vi "pcadctest.vi"() -> ()   [LabVIEW 2022 SP3]
uses:
  <vilib>/MakerHub/LINX/Public/Utilities/Open Serial.vi
  PCA/PCA.lvclass
  <vilib>/MakerHub/LINX/LMH-LINX.lvlib
panel:
  in  "Val 2 off":u16
  in  "Val off":u16
  in  "Val 3":u16=4095 format="%b"
  in  "Val 2":u16
  in  "Val":u16
  in  "GO":bool
  out "error out":errorcluster
  in  "stop":bool
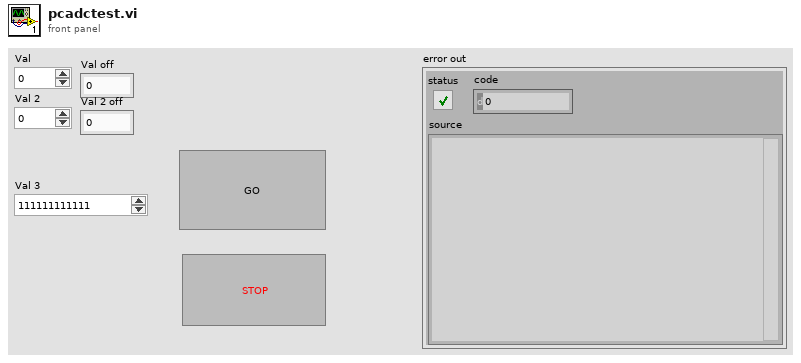
[diagram p1: front panel]
types:
  T1 = typedef "LMH-LINX.lvlib/LINX Ref.ctl" = cluster{"IO":T2, "Interface":T3, "LINX Device Config":T4}
  T2 = typedef "LMH-LINX.lvlib/Platform.ctl" = enum16{"Remote", "Local"}
  T3 = typedef "LMH-LINX.lvlib/Interface.ctl" = enum16{"Serial", "TCP"}
  T4 = typedef "LMH-LINX.lvlib/Device.lvlib/LINX Device Config.ctl" = cluster{"Interface":T3, "COM Port":refnum<visa-resource-name>, "TCP Configuration":T5, "Device Family":u8, "Device ID":u8, "Device Name":string, "TCP Ref":refnum<k5>, "Channels":T6}
  T5 = typedef "LMH-LINX.lvlib/Device.lvlib/TCP Config.ctl" = cluster{"IP Address":string, "Port":u16}
  T6 = typedef "LMH-LINX.lvlib/Channels.ctl" = cluster{"DI":u8[], "DO":u8[], "AI":u8[], "AO":u8[], "PWM":u8[], "QE":u8[], "UART":u8[], "I2C 2":u8[], "SPI":u8[], "CAN":u8[], "Servo":u8[], "AI Ref (V)":dbl, "AI Resolution (Bits)":u8, "AO Ref (V)":dbl, "AO Resolution (Bits)":u8}
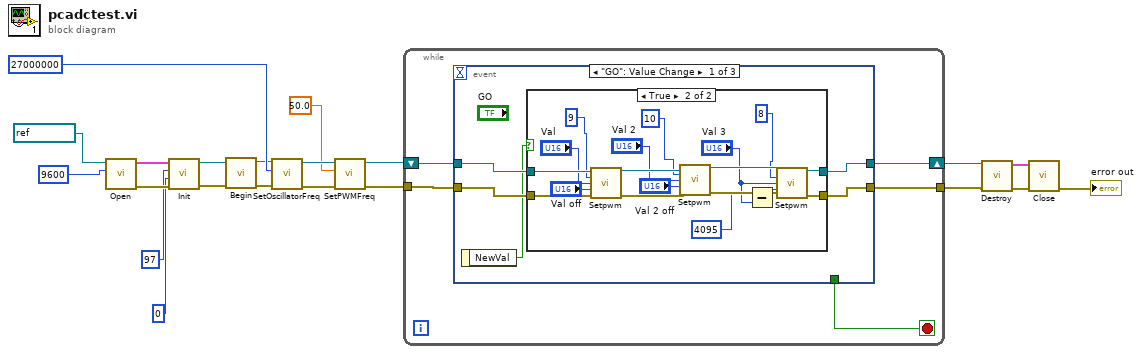
[diagram p0: block diagram]
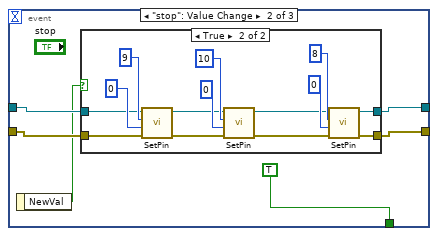
[diagram p3: hidden frame]
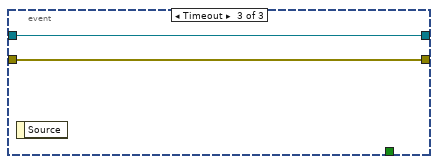
[diagram p5: hidden frame]
diagram:
  n1 = call-poly <vilib>:"Open.vi"("Baud Rate Override"=u32 9600, "Serial Port"=refnum<visa-resource-name> "COM4") -> ("Error Out"=w21:errorcluster, "LINX Resource"=w20:T1)  [unwired: 7 in, 1 out]
  n2 = call "Init.vi"("error in (no error)"=w21, "I2C Chanel(1)"=0, "I2C Slave Address (61)"=u16 97, "LINX Resource"=w20) -> ("error out"=w17:errorcluster, "PCA out"=w18:refnum<class "PCA.lvclass">)  [unwired: 6 in]
  n3 = call "Begin.vi"("error in (no error)"=w17, "PCA in"=w18) -> ("error out"=w16:errorcluster, "PCA out"=w15:refnum<class "PCA.lvclass">)  [unwired: 7 in, 1 out]
  n4 = call "SetOscillatorFreq.vi"("error in (no error)"=w16, "_oscillator_freq"=u32 27000000, "PCA in"=w15) -> ("error out"=w14:errorcluster, "PCA out"=w13:refnum<class "PCA.lvclass">)  [unwired: 7 in]
  n5 = call "SetPWMFreq.vi"("error in (no error)"=w14, "Freq"=sgl 50.0, "PCA in"=w13) -> ("error out"=w4:errorcluster, "PCA out"=w5:refnum<class "PCA.lvclass">)  [unwired: 7 in]
  n6 = while {
    tunnel: [w25] -> w12
    tunnel: w4 -> [w23]
    shift-right: [w24] -> w8
    shift-left: w5 -> [w26]
    stop <- w22 stop-if-true
    n7 = event shown="[0] \"GO\": Value Change" {
      selector: _ -> [_ _ _]
      dyn-events: _ -> [_ _ _]
      timeout: _ -> [_ _ _]
      tunnel: w26 -> [w31 w56 w74]
      tunnel: [w30 w54 w75] -> w25
      tunnel: [w29 w53 w74] -> w24
      tunnel: w23 -> [w28 w55 w75]
      tunnel: [_ TRUE _] -> w22
      event "GO": Value Change {
        n8 = event-data() -> ("NewVal"=w27:bool)  [unwired: 1 in]
        n9 = case shown="True" w27 {
          tunnel: w31 -> [w33 w47]
          tunnel: [w32 w44] -> w30
          tunnel: [w33 w45] -> w29
          tunnel: w28 -> [w32 w46]
          frame False {
          }
          frame True {
            n10 = call "Setpwm.vi"("PCA in"=w47, "Led num"=u8 9, "on"="Val", "off"="Val off", "error in (no error)"=w46) -> ("PCA out"=w51:refnum<class "PCA.lvclass">, "error out"=w50:errorcluster)  [unwired: 8 in, 1 out]
            n11 = call "Setpwm.vi"("PCA in"=w51, "Led num"=u8 10, "on"="Val 2", "off"="Val 2 off", "error in (no error)"=w50) -> ("PCA out"=w49:refnum<class "PCA.lvclass">, "error out"=w48:errorcluster)  [unwired: 8 in, 1 out]
            n12 = Subtract(x=u16 4095, y="Val 3") -> (x-y=w36:u16)
            n13 = call "Setpwm.vi"("PCA in"=w49, "Led num"=u8 8, "on"="Val 3", "off"=w36, "error in (no error)"=w48) -> ("PCA out"=w45:refnum<class "PCA.lvclass">, "error out"=w44:errorcluster)  [unwired: 8 in, 1 out]
          }
        }
      }
      event "stop": Value Change {
        n14 = event-data() -> ("NewVal"=w52:bool)  [unwired: 1 in]
        n15 = case shown="True" w52 {
          tunnel: w56 -> [w59 w63]
          tunnel: [w58 w62] -> w54
          tunnel: [w59 w61] -> w53
          tunnel: w55 -> [w58 w60]
          frame False {
          }
          frame True {
            n16 = call "SetPin.vi"("error in (no error)"=w60, "Val"=u16 0, "Led num"=u8 9, "PCA in"=w63) -> ("error out"=w68:errorcluster, "PCA out"=w69:refnum<class "PCA.lvclass">)  [unwired: 6 in]
            n17 = call "SetPin.vi"("error in (no error)"=w68, "Val"=u16 0, "Led num"=u8 10, "PCA in"=w69) -> ("error out"=w64:errorcluster, "PCA out"=w65:refnum<class "PCA.lvclass">)  [unwired: 6 in]
            n18 = call "SetPin.vi"("error in (no error)"=w64, "Val"=u16 0, "Led num"=u8 8, "PCA in"=w65) -> ("error out"=w62:errorcluster, "PCA out"=w61:refnum<class "PCA.lvclass">)  [unwired: 6 in]
          }
        }
      }
      event Timeout {
        n19 = event-data() -> ()  [unwired: 1 in, 1 out]
      }
    }
  }
  n20 = call "Destroy.vi"("error in (no error)"=w12, "PCA in"=w8) -> ("error out"=w11:errorcluster, "LINX Resource"=w10:T1)  [unwired: 8 in]
  n21 = call <vilib>:"Close.vi"("Error In"=w11, "LINX Resource"=w10) -> ("Error Out"=→"error out":errorcluster)  [unwired: 9 in]
